vi "初始设置.vi"(0 "引用句柄输入":refnum<k21>, 5 "error out":errorcluster caption="错误输出") -> (14 "task out":refnum<k21>, 19 "error IO":errorcluster)   [LabVIEW 2018]
uses:
  <vilib>/DAQmx/create/channels.llb/DAQmx Create Channel (AI-Sound Pressure-Microphone).vi
  <vilib>/DAQmx/configure/timing.llb/DAQmx Timing (Sample Clock).vi
  <resource>/objmgr/daqmx.rc
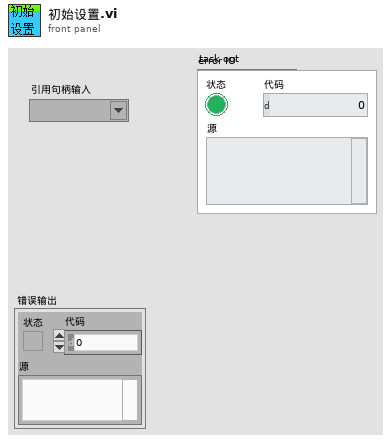
[diagram p1: front panel]
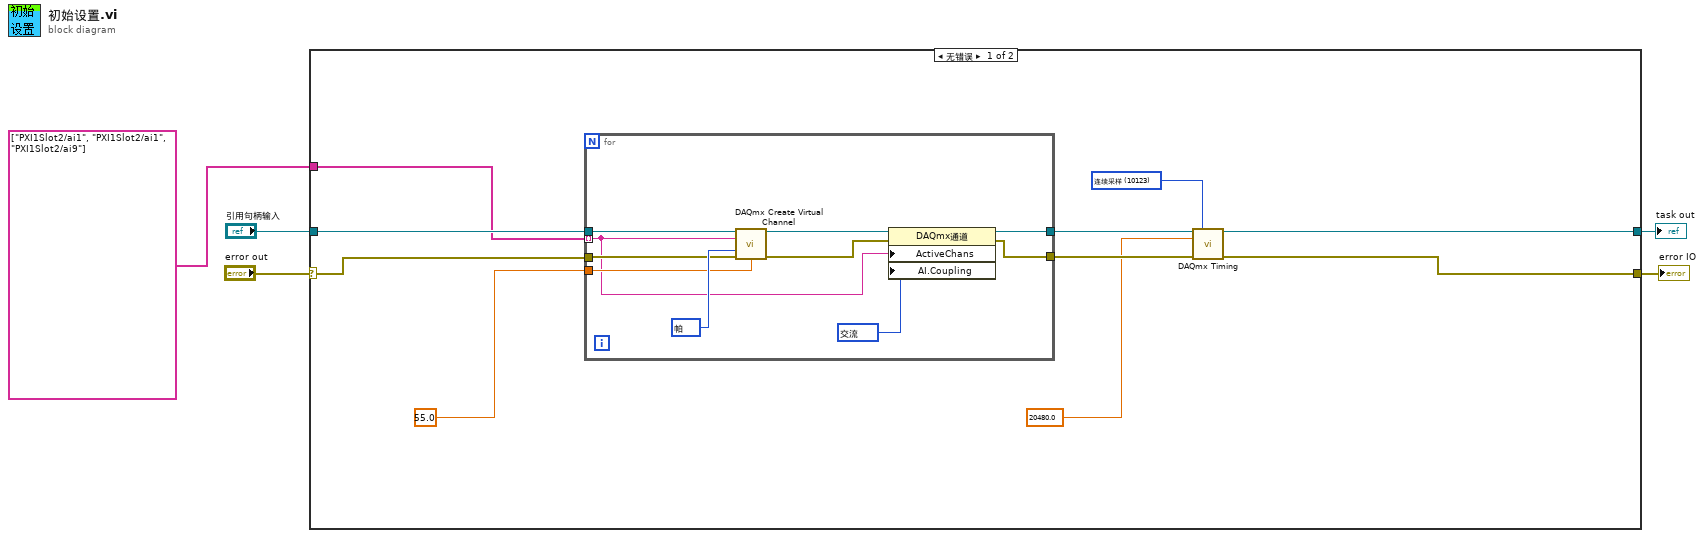
[diagram p0: block diagram]
diagram:
  n1 = case shown="无错误" "error out" {
    selector: "error out" -> [w14 w27]
    tunnel: "引用句柄输入" -> [w15 w26]
    tunnel: [w7 w26] -> w4
    tunnel: [w6 w27] -> w2
    tunnel: tag[] ["PXI1Slot2/ai1", "PXI1Slot2/ai1", "PXI1Slot2/ai9"] ("physical channels") -> [w9 _]
    frame No Error {
      w10 = 10123 items=["有限采样"=10178, "连续采样"=10123, "硬件定时单点"=12522] ("sample mode")
      n2 = for {
        tunnel: w9 -> [w16] mode=indexing
        tunnel: w15 -> [w24]
        tunnel: 55.0 -> [w23]
        tunnel: [w20] -> w13
        tunnel: [w18] -> w12
        tunnel: w14 -> [w22]
        w17 = 10045 items=["交流"=10045, "直流"=10050, "GND"=10066] ("AI.Coupling")
        w25 = 10081 items=["帕"=10081, "来自自定义换算"=10065] ("units")
        n3 = call-poly <vilib>:"DAQmx Create Virtual Channel.vi"("task in"=w24, "physical channels"=w16, "units"=w25, "error in"=w22, "microphone sensitivity"=w23) -> ("task out"=w21:refnum<k21>, "error out"=w19:errorcluster)  [unwired: 9 in]
        n4 = property class="DAQmx通道"(reference=w21, error in=w19, "ActiveChans"=w16, "AI.Coupling"=w17) -> (reference out=w20:refnum<k21>, error out=w18:errorcluster)
      }
      n5 = call-poly <vilib>:"DAQmx Timing.vi"("task/channels in"=w13, "sample mode"=w10, "rate"=20480.0, "error in"=w12) -> ("task out"=w7:refnum<k21>, "error out"=w6:errorcluster)  [unwired: 10 in]
    }
    frame Error {
    }
  }
  "task out" <- w4
  "error IO" <- w2
